vi "auto-drive-distance.vi"(4 "Acceleration (ft/s/s)":i32, 6 "Cruise Velocity (ft/s)":i32, 7 "Distance (ft)":dbl, 8 "Right Error In":errorcluster, 9 "Right Drive In":T1, 10 "Left Error In":errorcluster, 11 "Left Drive In":T1) -> (0 "Right Error Out":errorcluster, 1 "Right Drive Out":T1, 2 "Left Error Out":errorcluster, 3 "Left Drive Out":T1)   [LabVIEW 2019]
uses:
  <vilib>/Rock Robotics/WPI/ThirdParty/Phoenix-LabVIEW/Motor Controller/Controls/CTRE_Phoenix_MotorControl_ControlMode.ctl
  <vilib>/Rock Robotics/WPI/ThirdParty/Phoenix-LabVIEW/Motor Controller/Get/CTRE_Phoenix_MotorController_GetQuadratureData.vi
  <vilib>/Rock Robotics/SystemInterfaces/DIO/FPGA_DIOPWMChannel.ctl
  <vilib>/Rock Robotics/WPI/PWM/WPI_PWMDeadband.ctl
  <vilib>/Rock Robotics/WPI/MotorControl/WPI_MotorControlType.ctl
  <vilib>/Rock Robotics/SystemInterfaces/DIO/FPGA_DIOChannel.ctl
  <vilib>/Rock Robotics/WPI/MotorControl/WPI_MotorControlDeviceRef.ctl
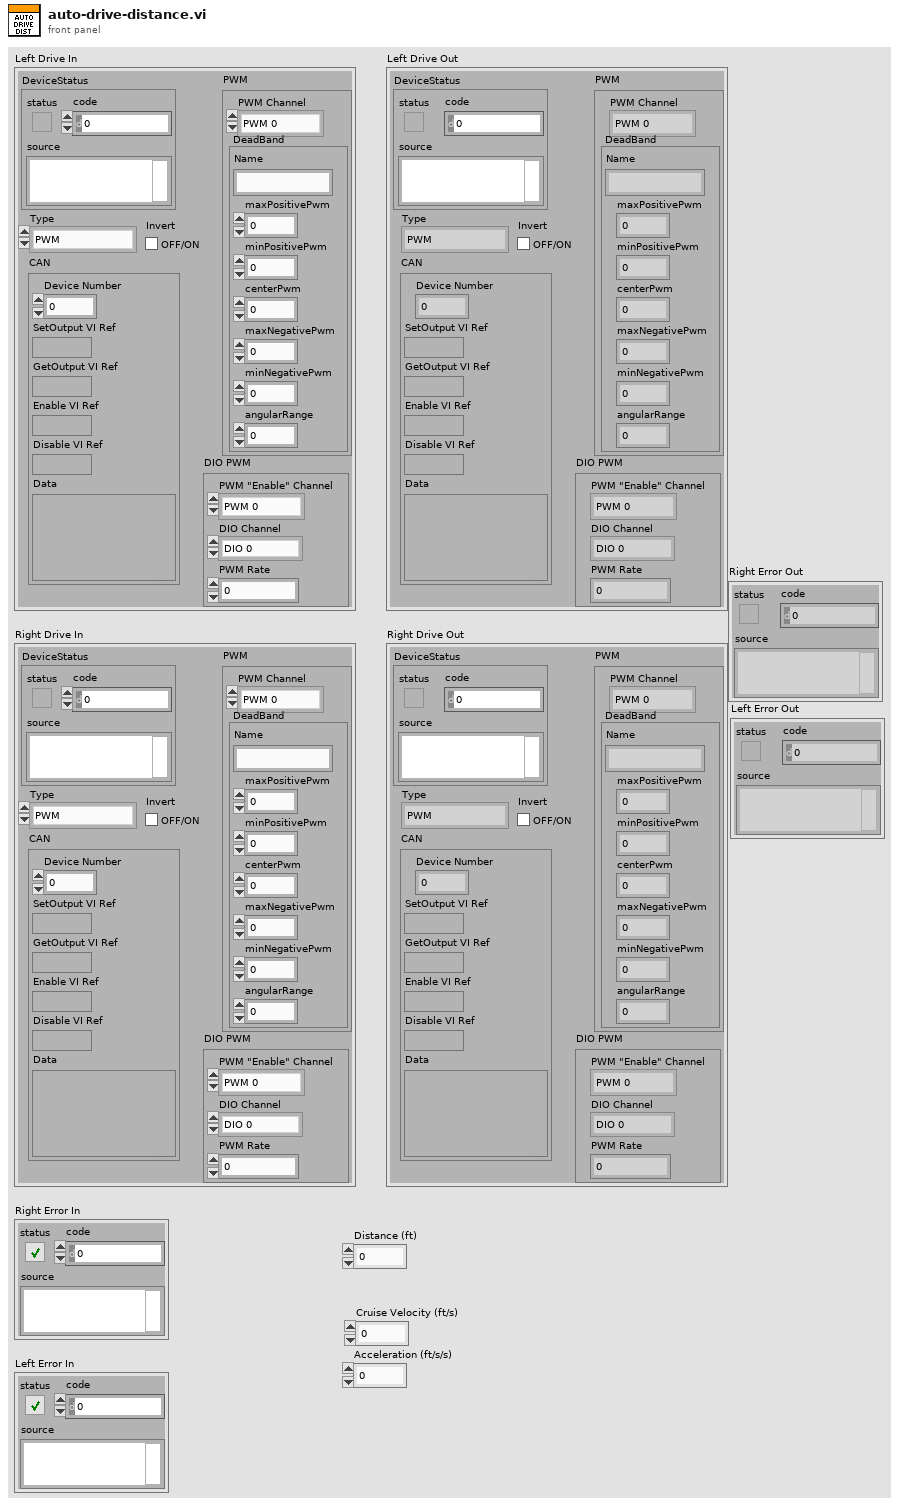
[diagram p1: front panel]
types:
  T1 = typedef "WPI_MotorControlDeviceRef.ctl" = cluster{"DeviceStatus":errorcluster, "Type":T2, "PWM":cluster{"PWM Channel":T3, "DeadBand":T4}, "CAN":cluster{"Device Number":u8, "SetOutput VI Ref":variant, "GetOutput VI Ref":variant, "Enable VI Ref":variant, "Disable VI Ref":variant, "Data":variant}, "Invert":bool, "DIO PWM":cluster{"PWM \"Enable\" Channel":T3, "DIOChannel":T5, "PWM Rate":dbl}}
  T2 = typedef "WPI_MotorControlType.ctl" = enum16{"PWM", "CAN", "DIO PWM"}
  T3 = typedef "FPGA_DIOPWMChannel.ctl" = enum8{"PWM 0", "PWM 1", "PWM 2", "PWM 3", "PWM 4", "PWM 5", "PWM 6", "PWM 7", "PWM 8", "PWM 9", "PWM MXP 0", "PWM MXP 1", "PWM MXP 2", "PWM MXP 3", "PWM MXP 4", "PWM MXP 5", "PWM MXP 6", "PWM MXP 7", "PWM MXP 8", "PWM MXP 9", "Invalid"}
  T4 = typedef "WPI_PWMDeadband.ctl" = cluster{"Name":string, "maxPositivePwm":i32, "minPositivePwm":i32, "centerPwm":i32, "maxNegativePwm":i32, "minNegativePwm":i32, "angularRange":u16}
  T5 = typedef "FPGA_DIOChannel.ctl" = enum8{"DIO 0", "DIO 1", "DIO 2", "DIO 3", "DIO 4", "DIO 5", "DIO 6", "DIO 7", "DIO 8", "DIO 9", "DIO MXP 0", "DIO MXP 1", "DIO MXP 2", "DIO MXP 3", "DIO MXP 4", "DIO MXP 5", "DIO MXP 6", "DIO MXP 7", "DIO MXP 8", "DIO MXP 9", "DIO MXP 10", "DIO MXP 11", "DIO MXP 12", "DIO MXP 13", "DIO MXP 14", "DIO MXP 15", "SPI Port CS1", "SPI Port CS2", "SPI Port CS3", "SPI Port MISO", "SPI Port MOSI", "Invalid"}
  T6 = typedef "CTRE_Phoenix_MotorControl_ControlMode.ctl" = u16
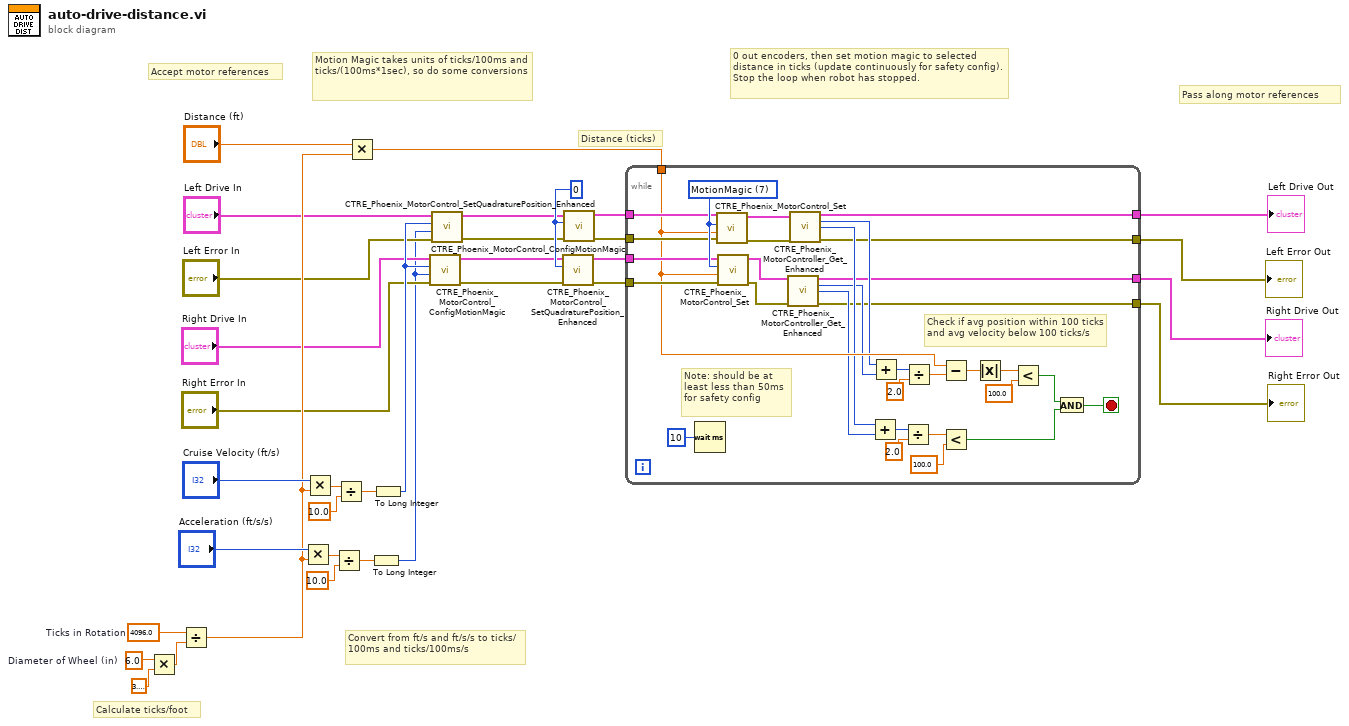
[diagram p0: block diagram]
diagram:
  w20 = 6.0  # Diameter of Wheel (in)
  w17 = 4096.0  # Ticks in Rotation
  w30 = 0 ("New Position")
  # "0 out encoders, then set motion magic to selected distance in ticks (update continuously for safety config). Stop the loop when robot has stopped."
  # "Distance (ticks)"
  # "Calculate ticks/foot"
  # "Convert from ft/s and ft/s/s to ticks/100ms and ticks/100ms/s"
  # "Accept motor references"
  # "Pass along motor references"
  # "Motion Magic takes units of ticks/100ms and ticks/(100ms*1sec), so do some conversions"
  n1 = Multiply(x=w20, y=3.141592653589793) -> (x*y=w24:dbl)
  n2 = Divide(x=w17, y=w24) -> (x/y=w15:dbl)
  n3 = Multiply(x="Acceleration (ft/s/s)", y=w15) -> (x*y=w22:dbl)
  n4 = Multiply(x="Cruise Velocity (ft/s)", y=w15) -> (x*y=w26:dbl)
  n5 = Divide(x=w22, y=10.0) -> (x/y=w23:dbl)
  n6 = Divide(x=w26, y=10.0) -> (x/y=w27:dbl)
  n7 = Multiply(x="Distance (ft)", y=w15) -> (x*y=w14:dbl)
  n8 = To Long Integer(number=w23) -> (32bit integer=w1:i32)
  n9 = To Long Integer(number=w27) -> (32bit integer=w28:i32)
  n10 = call <vilib>:"CTRE_Phoenix_MotorControl_ConfigMotionMagic.vi"("error in (no error)"="Right Error In", "Acceleration"=w1, "Cruise Velocity"=w28, "PhoenixMotorControlDevRef"="Right Drive In") -> ("error out"=w6:errorcluster, "PhoenixMotorControlDevRef"=w7:T1)  [unwired: 6 in]
  n11 = call <vilib>:"CTRE_Phoenix_MotorControl_ConfigMotionMagic.vi"("error in (no error)"="Left Error In", "Acceleration"=w1, "Cruise Velocity"=w28, "PhoenixMotorControlDevRef"="Left Drive In") -> ("error out"=w8:errorcluster, "PhoenixMotorControlDevRef"=w9:T1)  [unwired: 6 in]
  n12 = call <vilib>:"CTRE_Phoenix_MotorControl_SetQuadraturePosition_Enhanced.vi"("error in (no error)"=w6, "New Position"=w30, "PhoenixMotorControlDevRef"=w7) -> ("error out"=w34:errorcluster, "PhoenixMotorControlDevRef"=w33:T1)  [unwired: 7 in]
  n13 = call <vilib>:"CTRE_Phoenix_MotorControl_SetQuadraturePosition_Enhanced.vi"("error in (no error)"=w8, "New Position"=w30, "PhoenixMotorControlDevRef"=w9) -> ("error out"=w32:errorcluster, "PhoenixMotorControlDevRef"=w31:T1)  [unwired: 7 in]
  n14 = while {
    tunnel: w31 -> [w65]
    tunnel: w32 -> [w64]
    tunnel: w33 -> [w63]
    tunnel: w34 -> [w62]
    tunnel: w14 -> [w55]
    tunnel: [w38] -> w5
    tunnel: [w37] -> w4
    tunnel: [w36] -> w3
    tunnel: [w35] -> w2
    stop <- w50 stop-if-true
    w66 = T6 7 items=["PercentOutput"=0, "Position"=1, "Velocity"=2, "Current"=3, "Follower"=5, "MotionProfile"=6, "MotionMagic"=7, "MotionProfileArc"=10, "Disabled"=15] ("Control Mode")
    # "Note: should be at least less than 50ms for safety config"
    # "Check if avg position within 100 ticks and avg velocity below 100 ticks/s"
    n15 = Wait (ms)(milliseconds to wait=u32 10) -> ()  [unwired: 1 out]
    n16 = call <vilib>:"CTRE_Phoenix_MotorControl_Set.vi"("error in (no error)"=w64, "Output"=w55, "Control Mode"=w66, "PhoenixMotorControlDevRef"=w65) -> ("error out"=w45:errorcluster, "PhoenixMotorControlDevRef"=w46:T1)  [unwired: 6 in]
    n17 = call <vilib>:"CTRE_Phoenix_MotorControl_Set.vi"("error in (no error)"=w62, "Output"=w55, "Control Mode"=w66, "PhoenixMotorControlDevRef"=w63) -> ("error out"=w43:errorcluster, "PhoenixMotorControlDevRef"=w42:T1)  [unwired: 6 in]
    n18 = call-poly <vilib>:"CTRE_Phoenix_MotorController_Get_Enhanced.vi"("PhoenixMotorControlDevRef"=w42, "error in"=w43) -> ("PhoenixMotorControlDevRef"=w36:T1, "Quadrature Position"=w39:i32, "Quadrature Velocity"=w40:i32, "error out"=w35:errorcluster)  [unwired: 10 in]
    n19 = call-poly <vilib>:"CTRE_Phoenix_MotorController_Get_Enhanced.vi"("PhoenixMotorControlDevRef"=w46, "error in"=w45) -> ("PhoenixMotorControlDevRef"=w38:T1, "Quadrature Position"=w44:i32, "Quadrature Velocity"=w41:i32, "error out"=w37:errorcluster)  [unwired: 10 in]
    n20 = Add(x=w41, y=w40) -> (x+y=w59:i32)
    n21 = Add(x=w44, y=w39) -> (x+y=w61:i32)
    n22 = Divide(x=w59, y=2.0) -> (x/y=w49:dbl)
    n23 = Divide(x=w61, y=2.0) -> (x/y=w56:dbl)
    n24 = Subtract(x=w55, y=w56) -> (x-y=w54:dbl)
    n25 = Less?(x=w49, y=100.0) -> (x < y?=w47:bool)
    n26 = Absolute Value(x=w54) -> (abs(x)=w53:dbl)
    n27 = Less?(x=w53, y=100.0) -> (x < y?=w51:bool)
    n28 = And(x=w51, y=w47) -> (x .and. y?=w50:bool)
  }
  "Left Drive Out" <- w5
  "Right Drive Out" <- w3
  "Right Error Out" <- w2
  "Left Error Out" <- w4
